vi "Morphology (Erode).vi"(5 "Iterations (Default: 1)":u16=1, 7 "Anchor Point (Default -1,-1 Use Centre)":T2={"x"=-1, "y"=-1}, 8 "error in (no error)":errorcluster, 9 "Structuring Element":bool[][](array[boolean]), 10 "Morphology Result":T1, 11 "Greyscale Image-Source":T1) -> (0 "error out":errorcluster, 3 "Morphology Result (Duplicate)":T1)   [LabVIEW 2020, in "image.lvlib"]
uses:
  image.lvlib
  common/Image Point (Integer).ctl
  Greyscale Image.ctl
  MorphologyTypes.ctl
  common/Module Path.vi
  <vilib>/Utility/error.llb/Error Cluster From Error Code.vi
  common/common.lvlib
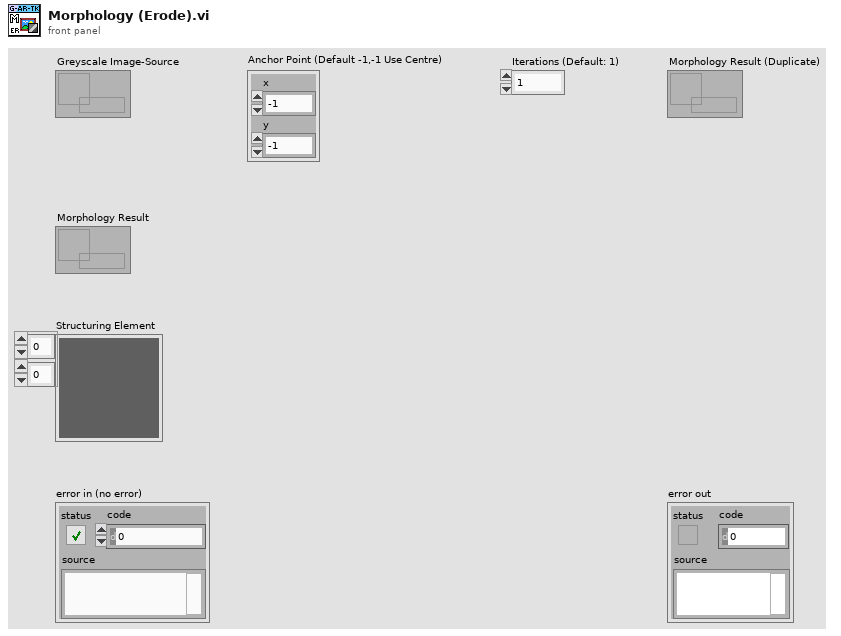
[diagram p1: front panel]
types:
  T1 = typedef "image.lvlib/Greyscale Image.ctl" = refnum<data-value>
  T2 = typedef "common.lvlib/Image Point (Integer).ctl" = cluster{"x":i32, "y":i32}
  T3 = typedef "image.lvlib/MorphologyTypes.ctl" = enum16{"MORPH_ERODE", "MORPH_DILATE", "MORPH_OPEN", "MORPH_CLOSE", "MORPH_GRADIENT", "MORPH_TOPHAT", "MORPH_BLACKHAT", "MORPH_HITMISS"}
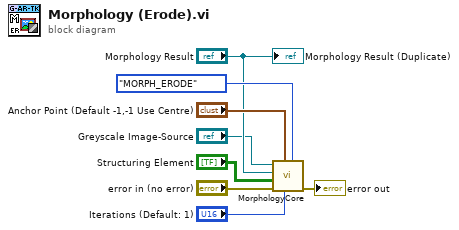
[diagram p0: block diagram]
diagram:
  n1 = call "MorphologyCore.vi"("MorphologyType"=MorphologyTypes."MORPH_ERODE", "Iterations"="Iterations (Default: 1)", "Anchor Point"="Anchor Point (Default -1,-1 Use Centre)", "error in (no error)"="error in (no error)", "Structuring Element"="Structuring Element", "Morphology Result"="Morphology Result", "Greyscale Image-Source"="Greyscale Image-Source") -> ("error out"=→"error out":errorcluster)  [unwired: 4 in]
  "Morphology Result (Duplicate)" <- "Morphology Result"
